vi "Timer FGV.vi"(7 "Mode":T1, 8 "error in (no error)":errorcluster, 11 "Timer Value (s)":dbl=1200.0 format="%#_13g") -> (0 "error out":errorcluster, 2 "Time Remaining (s)":dbl, 3 "Expired?":bool)   [LabVIEW 2020, in "MacroAssert.lvlib"]
doc: "FGV for setting, starting, and reading a timer."
uses:
  MacroAssert.lvlib
  CTLs/FGV Actions.ctl
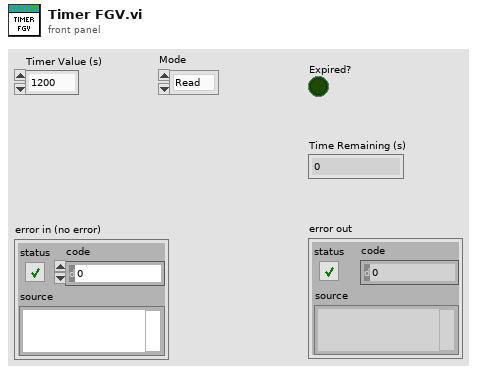
[diagram p1: front panel]
types:
  T1 = typedef "MacroAssert.lvlib/FGV Actions.ctl" = enum16{"Read", "Write"}
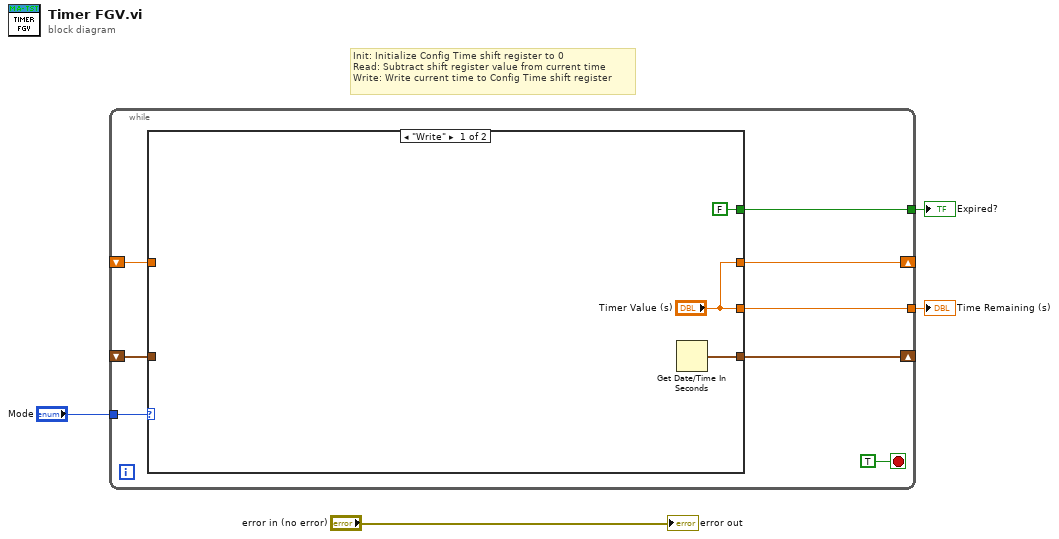
[diagram p0: block diagram]
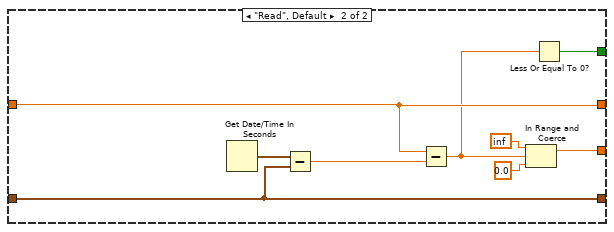
[diagram p2: hidden frame]
diagram:
  # "Init: Initialize Config Time shift register to 0\nRead: Subtract shift register value from current time\nWrite: Write current time to Config Time shift register"
  n1 = while {
    tunnel: "Mode" -> [w12]
    shift-right: [w10] -> _
    shift-left: _ -> [w11]
    tunnel: [w6] -> w2
    tunnel: [w8] -> w3
    shift-right: [w5] -> _
    shift-left: _ -> [w7]
    stop <- TRUE stop-if-true
    n2 = case shown="\"Write\"" w12 {
      tunnel: w11 -> [_ w23]
      tunnel: [w13 w23] -> w10
      tunnel: ["Timer Value (s)" w19] -> w8
      tunnel: w7 -> [_ w21]
      tunnel: [FALSE w22] -> w6
      tunnel: ["Timer Value (s)" w21] -> w5
      frame "Write" {
        n3 = Get Date/Time In Seconds() -> (seconds since 1Jan1904=w13:timestamp)
      }
      frame "Read", Default {
        n4 = Get Date/Time In Seconds() -> (seconds since 1Jan1904=w24:timestamp)
        n5 = Subtract(x=w24, y=w23) -> (x-y=w20:dbl)
        n6 = Subtract(x=w21, y=w20) -> (x-y=w16:dbl)
        n7 = In Range and Coerce(upper limit=inf, x=w16, lower limit=0.0) -> (coerced(x)=w19:dbl)  [unwired: 1 out]
        n8 = Less Or Equal To 0?(x=w16) -> (x <= 0?=w22:bool)
      }
    }
  }
  "Time Remaining (s)" <- w3
  "Expired?" <- w2
  "error out" <- "error in (no error)"
